vi "Read Adu Stream.vi"(7 "Timeout":u32, 8 "error in (no error)":errorcluster, 11 "Stream handle":u32) -> (0 "error out":errorcluster, 1 "Read Buffer":string, 2 "function return":i32, 3 "Stream handle out":u32)   [LabVIEW 2015, in "AduHid.lvlib"]
doc: "int __stdcall ReadAduStream(void * hStream,\n void * lpBuffer,\n unsigned long nNumberOfBytesToRead,\n unsigned long * lpNumberOfBytesRead,\n unsigned long iTimeout);"
uses:
  AduHid.lvlib
  Windows/SysWOW64/kernel32.dll
  AduHid.dll
panel:
  out "#BytesRead":u32
  in  "#BytesToRead":u32
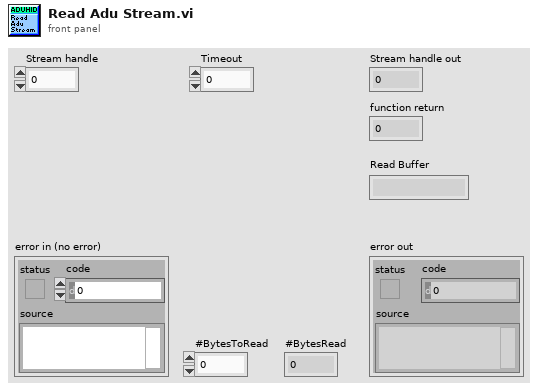
[diagram p1: front panel]
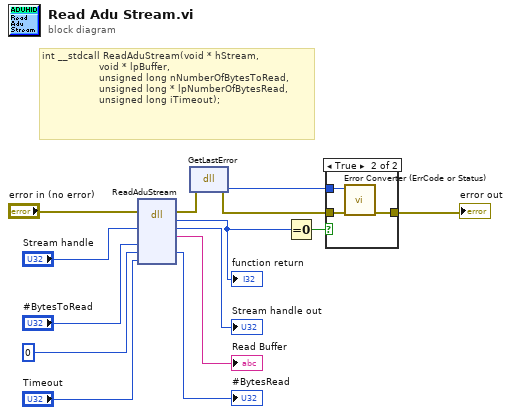
[diagram p0: block diagram]
diagram:
  # "int __stdcall ReadAduStream(void * hStream,\n                   void * lpBuffer,\n                   unsigned long nNumberOfBytesToRead,\n                   unsigned long * lpNumberOfBytesRead,\n                   unsigned long iTimeout);"
  n1 = dll-call lib="C:/Projects/CBTF Modules/Libraries/Ontrak ADU/API/AduHid.*" fn="ReadAduStream"(error in="error in (no error)", "Stream handle"="Stream handle", "#BytesToRead"="#BytesToRead", "#BytesRead"=u32 0, "Timeout"="Timeout") -> (error out=w3:errorcluster, "return type"=w2:i32, "Stream handle"=→"Stream handle out":u32, "Read Buffer"=→"Read Buffer":string, "#BytesRead"=→"#BytesRead":u32)  [unwired: 5 in, 1 out]
  "function return" <- w2
  n2 = dll-call lib="C:/Windows/SysWOW64/kernel32.dll" fn="GetLastError"(error in=w3) -> (error out=w6:errorcluster, "return type"=w5:u32)  [unwired: 2 in, 1 out]
  n3 = Equal To 0?(x=w2) -> (x = 0?=w4:bool)
  n4 = case shown="True" w4 {
    tunnel: [w15 w18] -> w1
    tunnel: w6 -> [w15 w17]
    tunnel: w5 -> [_ w16]
    frame False {
    }
    frame True {
      n5 = call "Error Converter (ErrCode or Status).vi"("error in (no error)"=w17, "last error"=w16) -> ("error out"=w18:errorcluster)  [unwired: 9 in]
    }
  }
  "error out" <- w1
